vi "quaternion_test.vi"() -> ()   [LabVIEW 2012]
panel:
  in  "stop":bool
  in  "Theta 2 degrees":dbl step=45.0
  in  "Theta 1 degrees":dbl step=45.0
  out "Q1 * QT * Q1'":dbl[](array[numeric])
  out "Q1 * Q2 theta":dbl format="%.5f"
  out "Q1 * Q2 axis":dbl[](array[numeric])
  out "Q1 * Q2 rotation":dbl[](array[numeric])
  in  "Test vector QT":dbl[](array[numeric])
  out "Rotation vector 1":dbl[](array[numeric])
  out "Theta 1 out":dbl format="%.5f"
  out "Axis 1 out":dbl[](array[numeric])
  out "Q2":dbl[](array[numeric])
  out "Q1":dbl[](array[numeric])
  out "Theta 2":dbl format="%.5f"
  in  "Axis 2":dbl[](array[numeric])
  in  "Axis 1":dbl[](array[numeric])
  out "Theta 1":dbl format="%.5f"
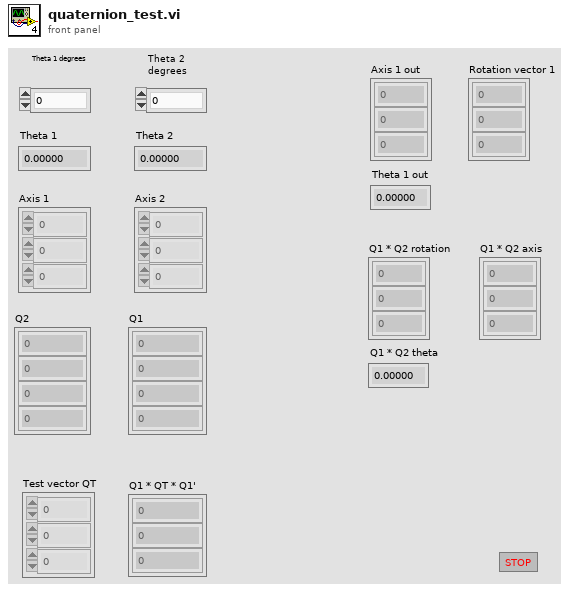
[diagram p1: front panel]
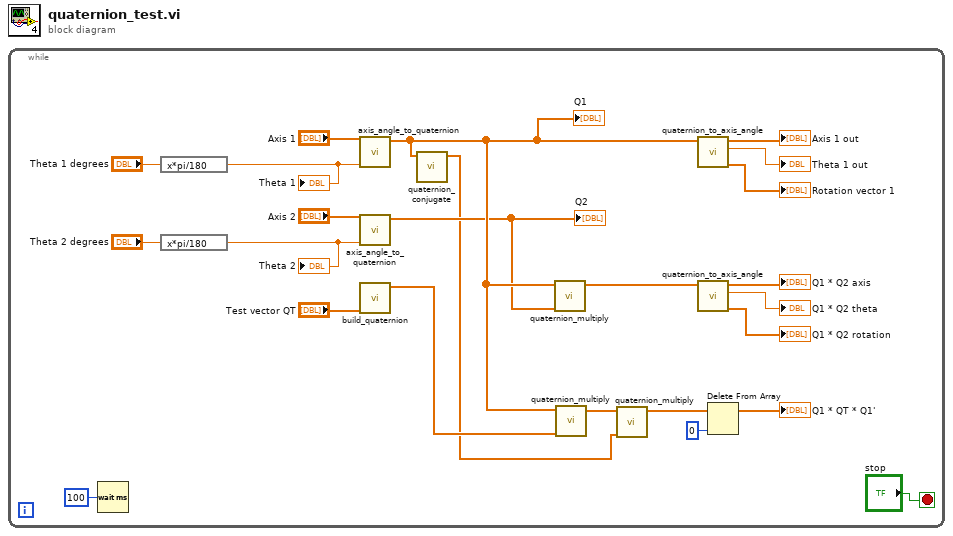
[diagram p0: block diagram]
diagram:
  n1 = while {
    stop <- "stop" stop-if-true
    n2 = Wait (ms)(milliseconds to wait=u32 100) -> ()  [unwired: 1 out]
    n3 = expression code="x*pi/180"("Theta 1 degrees") -> (w12:dbl)
    "Theta 1" <- w12
    n4 = expression code="x*pi/180"("Theta 2 degrees") -> (w11:dbl)
    "Theta 2" <- w11
    n5 = call "axis_angle_to_quaternion.vi"("Angle theta"=w12, "Axis x"="Axis 1") -> ("Quaternion"=w17:dbl[])  [unwired: 9 in]
    "Q1" <- w17
    n6 = call "axis_angle_to_quaternion.vi"("Angle theta"=w11, "Axis x"="Axis 2") -> ("Quaternion"=w15:dbl[])  [unwired: 9 in]
    "Q2" <- w15
    n7 = call "build_quaternion.vi"("x"="Test vector QT") -> ("Quaternion"=w9:dbl[])  [unwired: 10 in]
    n8 = call "quaternion_conjugate.vi"("Q"=w17) -> ("Q conjugate"=w8:dbl[])  [unwired: 10 in]
    n9 = call "quaternion_multiply.vi"("q2"=w15, "q1"=w17) -> ("q1 * q2"=w18:dbl[])  [unwired: 9 in]
    n10 = call "quaternion_multiply.vi"("q2"=w9, "q1"=w17) -> ("q1 * q2"=w16:dbl[])  [unwired: 9 in]
    n11 = call "quaternion_multiply.vi"("q2"=w8, "q1"=w16) -> ("q1 * q2"=w5:dbl[])  [unwired: 9 in]
    n12 = call "quaternion_to_axis_angle.vi"("Quaternion"=w17) -> ("Rotation vector"=→"Rotation vector 1":dbl[], "Angle theta"=→"Theta 1 out":dbl, "Axis x"=→"Axis 1 out":dbl[])  [unwired: 8 in]
    n13 = call "quaternion_to_axis_angle.vi"("Quaternion"=w18) -> ("Rotation vector"=→"Q1 * Q2 rotation":dbl[], "Angle theta"=→"Q1 * Q2 theta":dbl, "Axis x"=→"Q1 * Q2 axis":dbl[])  [unwired: 8 in]
    n14 = Delete From Array(array=w5, index=0) -> (array with subset deleted=→"Q1 * QT * Q1'":dbl[])  [unwired: 1 in, 1 out]
  }
